vi "pic_Zoom (interpolayciay po blijaishemu sosedu).vi"(2 "Zoom":dbl=1.5 format="%#_1g", 3 "image data IN":T1) -> (1 "image data OUT":T1)   [LabVIEW 2018]
uses:
  <vilib>/picture/picture.llb/imagedata.ctl
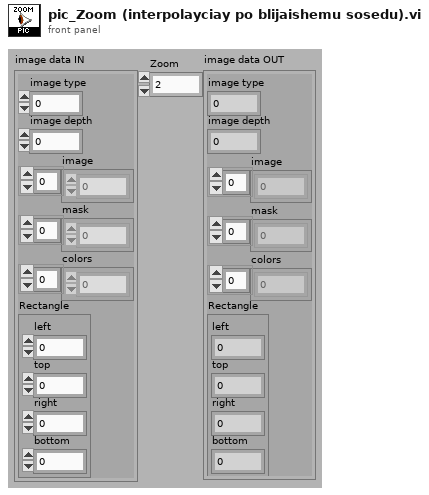
[diagram p1: front panel]
types:
  T1 = typedef "imagedata.ctl" = cluster{"image type":i32, "image depth":i32, "image":u8[], "mask":u8[], "colors":u32[], "Rectangle":cluster{"left":i16, "top":i16, "right":i16, "bottom":i16}}
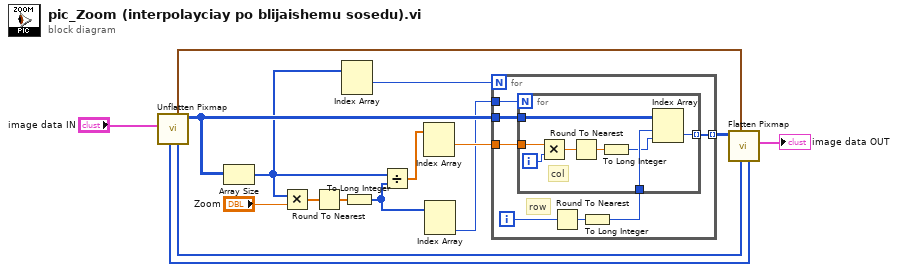
[diagram p0: block diagram]
diagram:
  n1 = call <vilib>:"Unflatten Pixmap.vi"("image data"="image data IN") -> ("24-bit pixmap"=w9:u32[][], "colors"=w7:u32[], "top left"=w5:cluster{"x":i16, "y":i16}, "mask"=w6:u8[])  [unwired: 7 out]
  n2 = Array Size(array=w9) -> (size(s)=w2:i32[])
  n3 = Multiply(x=w2, y="Zoom") -> (x*y=w14:dbl[])
  n4 = Round To Nearest(number=w14) -> (nearest integer value=w13:dbl[])
  n5 = Index Array(array=w2) -> (element #1=w1:i32)  [unwired: 2 in, 1 out]
  n6 = To Long Integer(number=w13) -> (32bit integer=w12:i32[])
  n7 = Divide(x=w2, y=w12) -> (x/y=w11:dbl[])
  n8 = Index Array(array=w11) -> (element #1=w10:dbl)  [unwired: 2 in, 1 out]
  n9 = Index Array(array=w12) -> (element #2=w3:i32)  [unwired: 2 in, 1 out]
  n10 = for {
    N: w1 -> [_]
    tunnel: w3 -> [w23]
    tunnel: w10 -> [w22]
    tunnel: w9 -> [w20]
    tunnel: [w18] -> w8 mode=indexing
    i -> [w17]
    # "row"
    n11 = Round To Nearest(number=w17) -> (nearest integer value=w21:i32)
    n12 = To Long Integer(number=w21) -> (32bit integer=w19:i32)
    n13 = for {
      N: w23 -> [_]
      tunnel: w22 -> [w30]
      tunnel: w20 -> [w27]
      tunnel: w19 -> [w25]
      tunnel: [w26] -> w18 mode=indexing
      i -> [w31]
      # "col"
      n14 = Multiply(x=w30, y=w31) -> (x*y=w28:dbl)
      n15 = Round To Nearest(number=w28) -> (nearest integer value=w29:dbl)
      n16 = To Long Integer(number=w29) -> (32bit integer=w24:i32)
      n17 = Index Array(array=w27, index (row)=w25, index (col)=w24) -> (element=w26:u32)
    }
  }
  n18 = call <vilib>:"Flatten Pixmap.vi"("mask"=w6, "colors"=w7, "top left"=w5, "24-bit pixmap"=w8) -> ("image data"=→"image data OUT":T1)  [unwired: 3 in, 4 out]
